vi "RANGE Write To File.vi"(6 "Time":dbl, 8 "Error In":errorcluster, 9 "All Meter Data":T2={"Meter 1"={"Meter Size"=0.0, "DAQ Output (Voltage)"=0.0, "Reference (Voltage)"=0.0, "Meter Present"=FALSE, "Meter Visa"="COM3", "Gas Type"="", "SLPM Error @ Zero"=0.0, "Gas Mix Number"="", "Set STP Register"=FALSE, "Measurement Units"={"Abs. Pressure"="", "Gauge/Diff. Press."="", "Barometric Press."="", "Temperature"="", "Volume"="", "Mass"="", "Setpoint"="", "Valve Drive"="", "Totalizer"="", "Tot. Timer"="", "Tot. Avg. Flow"="", "Tot. Peak Flow"="", "Software Version"=""}}, "Meter 2"={"Meter Size"=0.0, "DAQ Output (Voltage)"=0.0, "Reference (Voltage)"=0.0, "Meter Present"=FALSE, "Meter Visa"="COM3", "Gas Type"="", "SLPM Error @ Zero"=0.0, "Gas Mix Number"="", "Set STP Register"=FALSE, "Measurement Units"={"Abs. Pressure"="", "Gauge/Diff. Press."="", "Barometric Press."="", "Temperature"="", "Volume"="", "Mass"="", "Setpoint"="", "Valve Drive"="", "Totalizer"="", "Tot. Timer"="", "Tot. Avg. Flow"="", "Tot. Peak Flow"="", "Software Version"=""}}, "Meter 3"={"Meter Size"=0.0, "DAQ Output (Voltage)"=0.0, "Reference (Voltage)"=0.0, "Meter Present"=FALSE, "Meter Visa"="COM3", "Gas Type"="", "SLPM Error @ Zero"=0.0, "Gas Mix Number"="", "Set STP Register"=FALSE, "Measurement Units"={"Abs. Pressure"="", "Gauge/Diff. Press."="", "Barometric Press."="", "Temperature"="", "Volume"="", "Mass"="", "Setpoint"="", "Valve Drive"="", "Totalizer"="", "Tot. Timer"="", "Tot. Avg. Flow"="", "Tot. Peak Flow"="", "Software Version"=""}}, "Meter 4"={"Meter Size"=0.0, "DAQ Output (Voltage)"=0.0, "Reference (Voltage)"=0.0, "Meter Present"=FALSE, "Meter Visa"="COM3", "Gas Type"="", "SLPM Error @ Zero"=0.0, "Gas Mix Number"="", "Set STP Register"=FALSE, "Measurement Units"={"Abs. Pressure"="", "Gauge/Diff. Press."="", "Barometric Press."="", "Temperature"="", "Volume"="", "Mass"="", "Setpoint"="", "Valve Drive"="", "Totalizer"="", "Tot. Timer"="", "Tot. Avg. Flow"="", "Tot. Peak Flow"="", "Software Version"=""}}, "Meter 5"={"Meter Size"=0.0, "DAQ Output (Voltage)"=0.0, "Reference (Voltage)"=0.0, "Meter Present"=FALSE, "Meter Visa"="COM3", "Gas Type"="", "SLPM Error @ Zero"=0.0, "Gas Mix Number"="", "Set STP Register"=FALSE, "Measurement Units"={"Abs. Pressure"="", "Gauge/Diff. Press."="", "Barometric Press."="", "Temperature"="", "Volume"="", "Mass"="", "Setpoint"="", "Valve Drive"="", "Totalizer"="", "Tot. Timer"="", "Tot. Avg. Flow"="", "Tot. Peak Flow"="", "Software Version"=""}}, "Meter 6"={"Meter Size"=0.0, "DAQ Output (Voltage)"=0.0, "Reference (Voltage)"=0.0, "Meter Present"=FALSE, "Meter Visa"="COM3", "Gas Type"="", "SLPM Error @ Zero"=0.0, "Gas Mix Number"="", "Set STP Register"=FALSE, "Measurement Units"={"Abs. Pressure"="", "Gauge/Diff. Press."="", "Barometric Press."="", "Temperature"="", "Volume"="", "Mass"="", "Setpoint"="", "Valve Drive"="", "Totalizer"="", "Tot. Timer"="", "Tot. Avg. Flow"="", "Tot. Peak Flow"="", "Software Version"=""}}, "Meter Bank 1"={"Flow Rate (BTU/HR)"=0.0, "ANSI Placeholder Array"=[], "15 Sec Avg Array"=[], "30 Sec Avg Array "=[], "ANSI Average (BTU/HR)"=0.0, "Panel Data"={"Meter Type (Gas)"="", "Heating Value (BTU/ft³)"=0.0, "Ft³ / Hr (SCFH)"=0.0, "15 Second Average (BTU/HR)"=0.0, "30 Second Average (BTU/HR)"=0.0, "Mass Flow"=0.0, "Vol. Flow"=0.0, "Gas Temperature"=0.0, "Gas Pressure"=0.0, "Tot.Flow"=0.0}, "Start ANSI"=FALSE, "ANSI Start Time"=0.0, "Restart ANSI"=FALSE, "Meter ID"=""}, "Meter Bank 2"={"Flow Rate (BTU/HR)"=0.0, "ANSI Placeholder Array"=[], "15 Sec Avg Array"=[], "30 Sec Avg Array "=[], "ANSI Average (BTU/HR)"=0.0, "Panel Data"={"Meter Type (Gas)"="", "Heating Value (BTU/ft³)"=0.0, "Ft³ / Hr (SCFH)"=0.0, "15 Second Average (BTU/HR)"=0.0, "30 Second Average (BTU/HR)"=0.0, "Mass Flow"=0.0, "Vol. Flow"=0.0, "Gas Temperature"=0.0, "Gas Pressure"=0.0, "Tot.Flow"=0.0}, "Start ANSI"=FALSE, "ANSI Start Time"=0.0, "Restart ANSI"=FALSE, "Meter ID"=""}, "Meter Bank 3"={"Flow Rate (BTU/HR)"=0.0, "ANSI Placeholder Array"=[], "15 Sec Avg Array"=[], "30 Sec Avg Array "=[], "ANSI Average (BTU/HR)"=0.0, "Panel Data"={"Meter Type (Gas)"="", "Heating Value (BTU/ft³)"=0.0, "Ft³ / Hr (SCFH)"=0.0, "15 Second Average (BTU/HR)"=0.0, "30 Second Average (BTU/HR)"=0.0, "Mass Flow"=0.0, "Vol. Flow"=0.0, "Gas Temperature"=0.0, "Gas Pressure"=0.0, "Tot.Flow"=0.0}, "Start ANSI"=FALSE, "ANSI Start Time"=0.0, "Restart ANSI"=FALSE, "Meter ID"=""}, "Threshold Voltage (NI DAQ)"=0.2, "Use RS232 Data Collection"=FALSE, "Use Auto Switching"=FALSE}, 11 "File Path":path) -> (0 "Error Out":errorcluster)   [LabVIEW 2016]
uses:
  Type Definitions/RANGE DAQ Data Four Meters.ctl
  Type Definitions/RANGE DAQ Data.ctl
  Drivers/Omega FMA-1600A Series Gas Flow Meter/Type Definitions/FMA1600A Gas Type.ctl
  Drivers/Omega FMA-1600A Series Gas Flow Meter/Type Definitions/FMA1600A Units String.ctl
  Type Definitions/RANGE GAS Data.ctl
  Type Definitions/RANGE Panel Data.ctl
  <vilib>/Utility/file.llb/Write Delimited Spreadsheet (string).vi
panel:
  out "Debug":T1[](array[typedef])
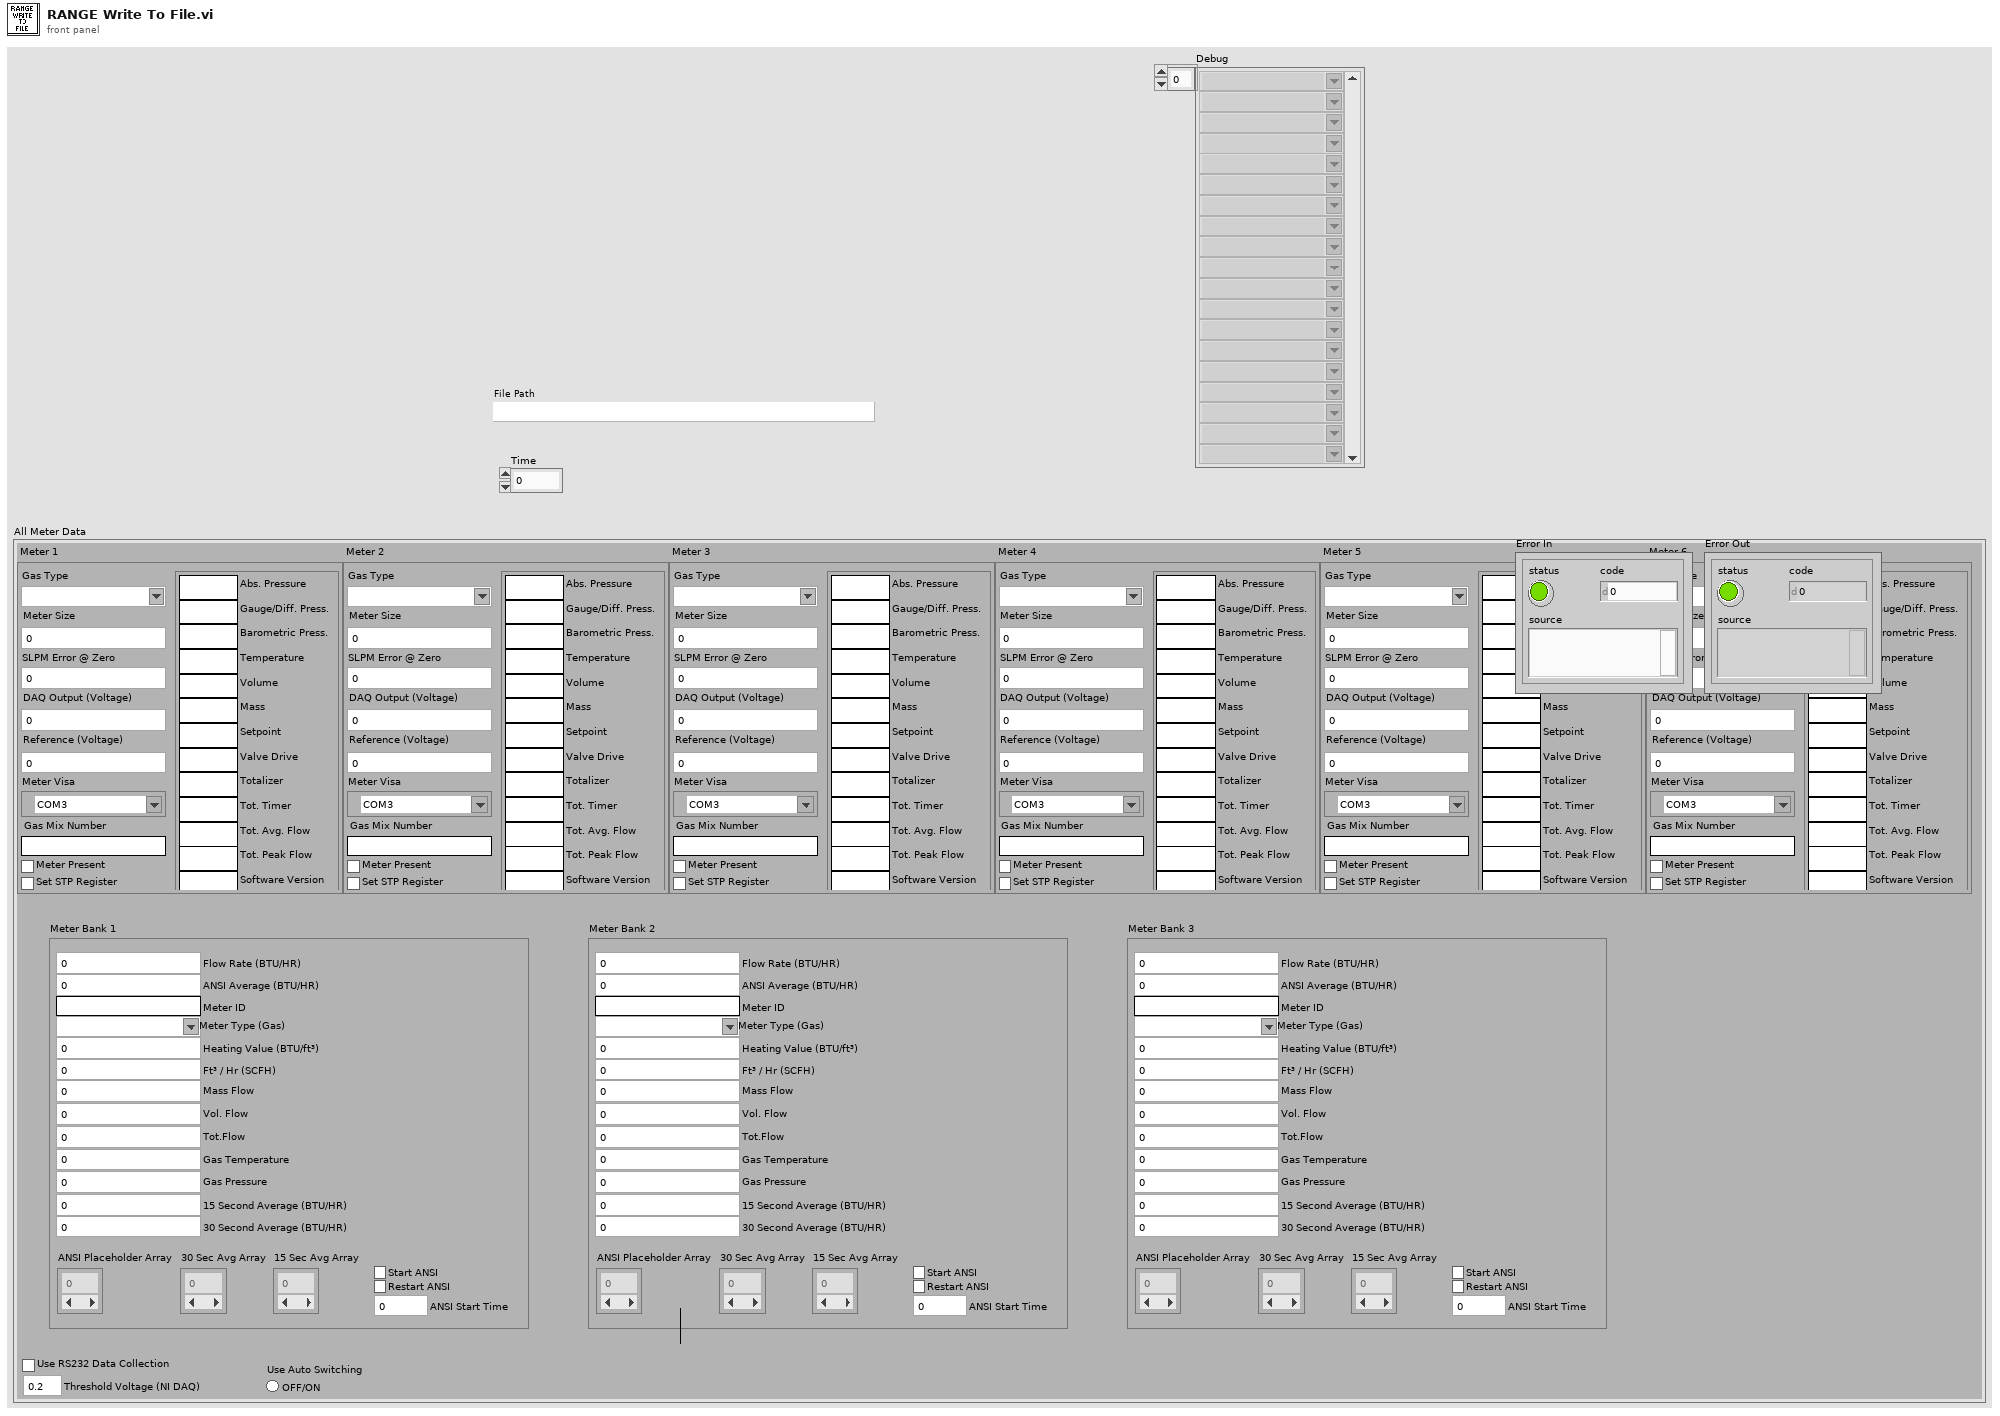
[diagram p1: front panel]
types:
  T1 = typedef "FMA1600A Gas Type.ctl" = string
  T2 = typedef "RANGE DAQ Data Four Meters.ctl" = cluster{"Meter 1":T3, "Meter 2":T3, "Meter 3":T3, "Meter 4":T3, "Meter 5":T3, "Meter 6":T3, "Meter Bank 1":T5, "Meter Bank 2":T5, "Meter Bank 3":T5, "Threshold Voltage (NI DAQ)":dbl, "Use RS232 Data Collection":bool, "Use Auto Switching":bool}
  T3 = typedef "RANGE DAQ Data.ctl" = cluster{"Meter Size":dbl, "DAQ Output (Voltage)":dbl, "Reference (Voltage)":dbl, "Meter Present":bool, "Meter Visa":refnum<visa-resource-name>, "Gas Type":T1, "SLPM Error @ Zero":dbl, "Gas Mix Number":string, "Set STP Register":bool, "Measurement Units":T4}
  T4 = typedef "FMA1600A Units String.ctl" = cluster{"Abs. Pressure":string, "Gauge/Diff. Press.":string, "Barometric Press.":string, "Temperature":string, "Volume":string, "Mass":string, "Setpoint":string, "Valve Drive":string, "Totalizer":string, "Tot. Timer":string, "Tot. Avg. Flow":string, "Tot. Peak Flow":string, "Software Version":string}
  T5 = typedef "RANGE GAS Data.ctl" = cluster{"Flow Rate (BTU/HR)":dbl, "ANSI Placeholder Array":dbl[], "15 Sec Avg Array":dbl[], "30 Sec Avg Array ":dbl[], "ANSI Average (BTU/HR)":dbl, "Panel Data":T6, "Start ANSI":bool, "ANSI Start Time":dbl, "Restart ANSI":bool, "Meter ID":string}
  T6 = typedef "RANGE Panel Data.ctl" = cluster{"Meter Type (Gas)":T1, "Heating Value (BTU/ft³)":dbl, "Ft³ / Hr (SCFH)":dbl, "15 Second Average (BTU/HR)":dbl, "30 Second Average (BTU/HR)":dbl, "Mass Flow":dbl, "Vol. Flow":dbl, "Gas Temperature":dbl, "Gas Pressure":dbl, "Tot.Flow":dbl}
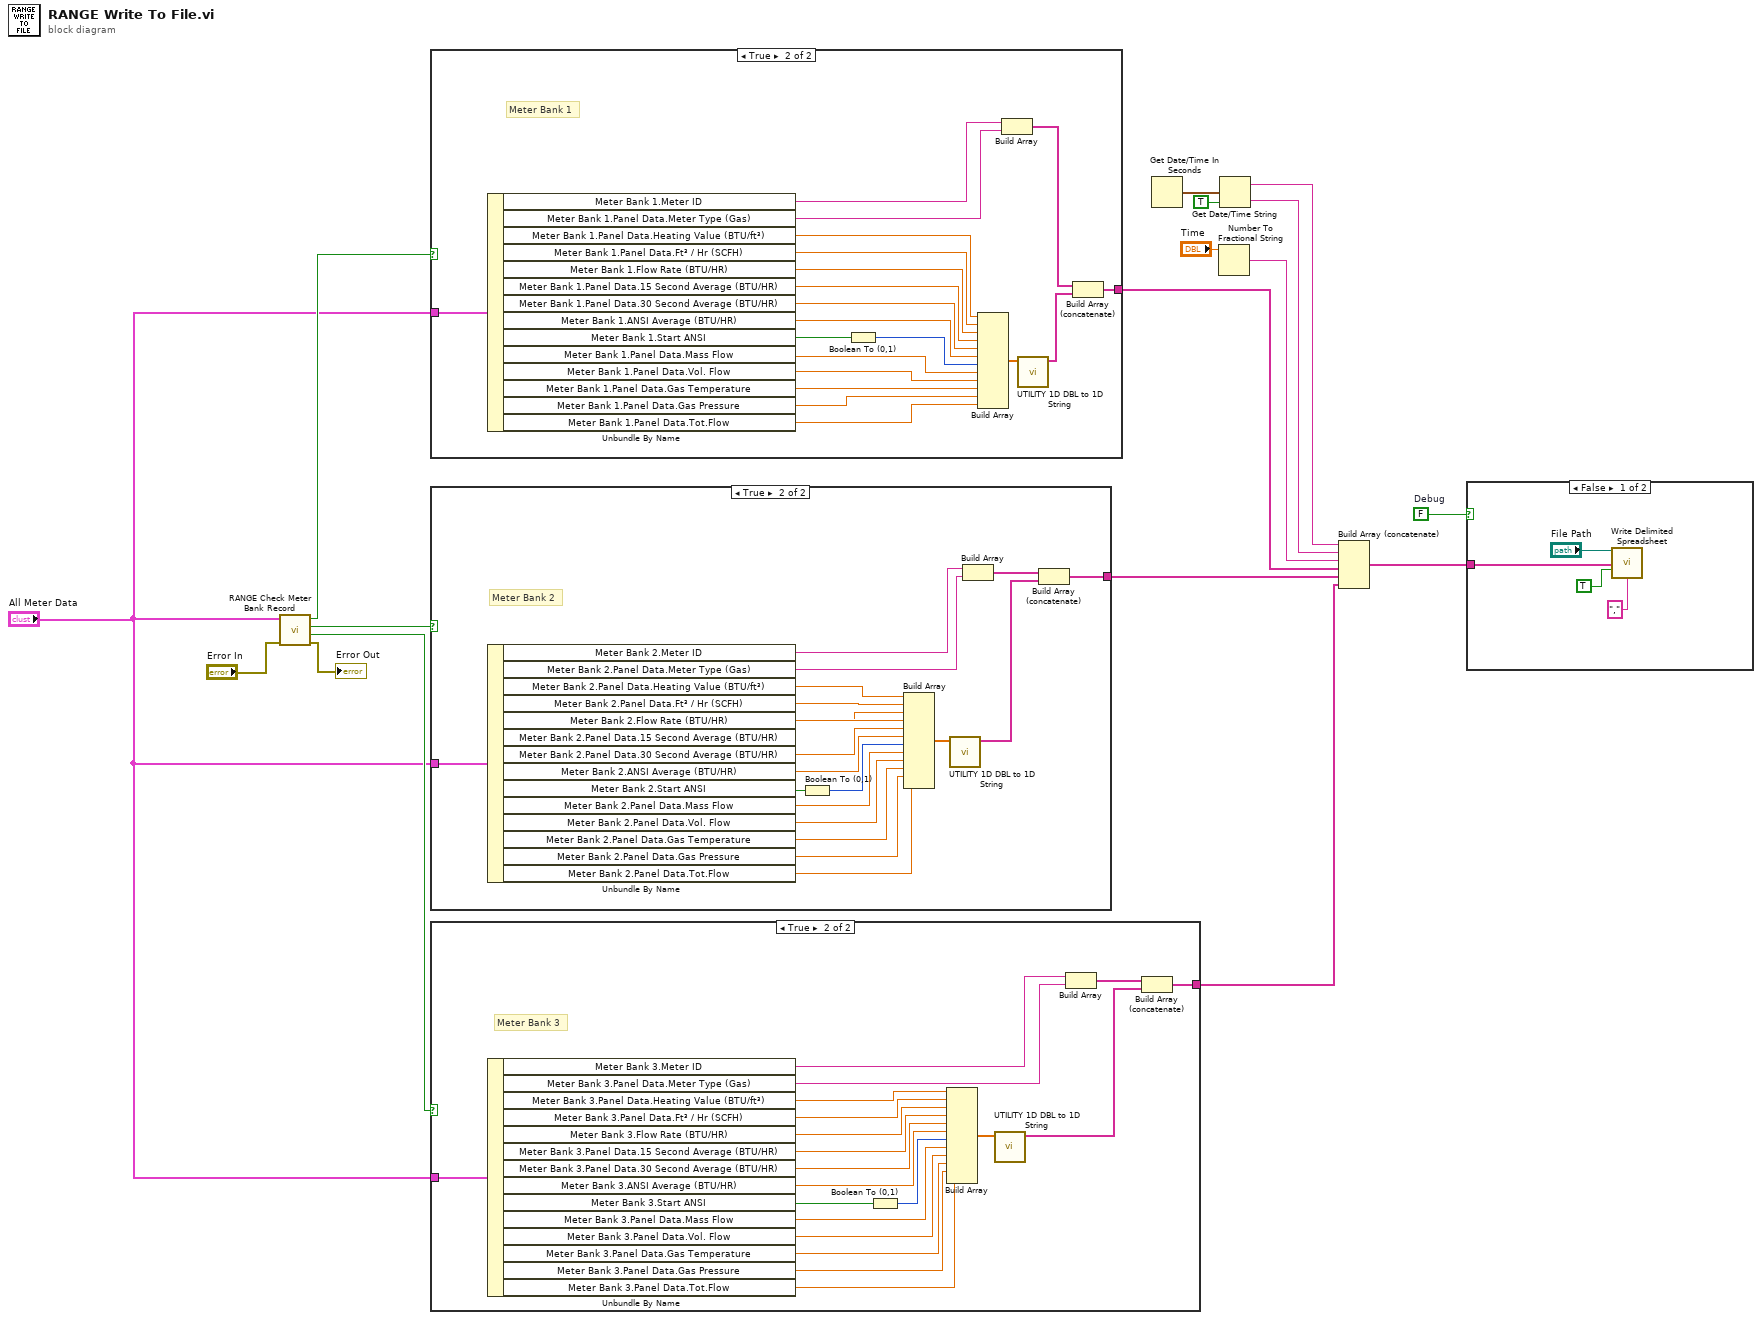
[diagram p0: block diagram]
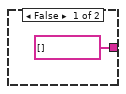
[diagram p2: hidden frame]
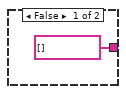
[diagram p3: hidden frame]
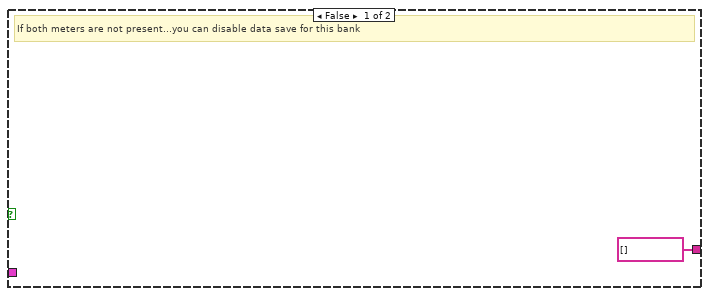
[diagram p4: hidden frame]
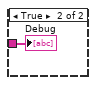
[diagram p5: hidden frame]
diagram:
  w7 = FALSE  # Debug
  n1 = call "RANGE Check Meter Bank Record.vi"("Error In"="Error In", "All Meter Data"="All Meter Data") -> ("Error Out"=→"Error Out":errorcluster, "Meter Bank 3"=w4:bool, "Meter Bank 2"=w5:bool, "Meter Bank 1"=w6:bool)  [unwired: 6 in]
  n2 = case shown="True" w6 {
    tunnel: "All Meter Data" -> [_ w31]
    tunnel: [T1[] [] w21] -> w15
    frame False {
      # "If both meters are not present...you can disable data save for this bank"
    }
    frame True {
      # "Meter Bank 1"
      n3 = Unbundle By Name(w31) -> ("Meter Bank 1.Meter ID"=w19:string, "Meter Bank 1.Panel Data.Meter Type (Gas)"=w24:T1, "Meter Bank 1.Panel Data.Heating Value (BTU/ft³)"=w38:dbl, "Meter Bank 1.Panel Data.Ft³ / Hr (SCFH)"=w37:dbl, "Meter Bank 1.Flow Rate (BTU/HR)"=w36:dbl, "Meter Bank 1.Panel Data.15 Second Average (BTU/HR)"=w35:dbl, "Meter Bank 1.Panel Data.30 Second Average (BTU/HR)"=w34:dbl, "Meter Bank 1.ANSI Average (BTU/HR)"=w33:dbl, "Meter Bank 1.Start ANSI"=w30:bool, "Meter Bank 1.Panel Data.Mass Flow"=w29:dbl, "Meter Bank 1.Panel Data.Vol. Flow"=w28:dbl, "Meter Bank 1.Panel Data.Gas Temperature"=w27:dbl, "Meter Bank 1.Panel Data.Gas Pressure"=w26:dbl, "Meter Bank 1.Panel Data.Tot.Flow"=w20:dbl)
      n4 = Boolean To (0,1)(Boolean=w30) -> (0, 1=w32:i16)
      n5 = Build Array(w38, w37, w36, w35, w34, w33, w32, w29, w28, w27, w26, w20) -> (w25:dbl[])
      n6 = Build Array(w19, w24) -> (w22:T1[])
      n7 = call "UTILITY 1D DBL to 1D String.vi"("1D DBL"=w25) -> ("1D String"=w23:string[])  [unwired: 10 in]
      n8 = Build Array (concatenate)(w22, w23) -> (w21:T1[])
    }
  }
  n9 = case shown="True" w5 {
    tunnel: [T1[] [] w43] -> w14
    tunnel: "All Meter Data" -> [_ w41]
    frame False {
    }
    frame True {
      # "Meter Bank 2"
      n10 = Unbundle By Name(w41) -> ("Meter Bank 2.Meter ID"=w40:string, "Meter Bank 2.Panel Data.Meter Type (Gas)"=w46:T1, "Meter Bank 2.Panel Data.Heating Value (BTU/ft³)"=w54:dbl, "Meter Bank 2.Panel Data.Ft³ / Hr (SCFH)"=w55:dbl, "Meter Bank 2.Flow Rate (BTU/HR)"=w56:dbl, "Meter Bank 2.Panel Data.15 Second Average (BTU/HR)"=w57:dbl, "Meter Bank 2.Panel Data.30 Second Average (BTU/HR)"=w58:dbl, "Meter Bank 2.ANSI Average (BTU/HR)"=w59:dbl, "Meter Bank 2.Start ANSI"=w52:bool, "Meter Bank 2.Panel Data.Mass Flow"=w51:dbl, "Meter Bank 2.Panel Data.Vol. Flow"=w50:dbl, "Meter Bank 2.Panel Data.Gas Temperature"=w49:dbl, "Meter Bank 2.Panel Data.Gas Pressure"=w48:dbl, "Meter Bank 2.Panel Data.Tot.Flow"=w42:dbl)
      n11 = Boolean To (0,1)(Boolean=w52) -> (0, 1=w53:i16)
      n12 = Build Array(w54, w55, w56, w57, w58, w59, w53, w51, w50, w49, w48, w42) -> (w47:dbl[])
      n13 = call "UTILITY 1D DBL to 1D String.vi"("1D DBL"=w47) -> ("1D String"=w45:string[])  [unwired: 10 in]
      n14 = Build Array(w40, w46) -> (w44:T1[])
      n15 = Build Array (concatenate)(w44, w45) -> (w43:T1[])
    }
  }
  n16 = case shown="True" w4 {
    tunnel: [T1[] [] w64] -> w13
    tunnel: "All Meter Data" -> [_ w62]
    frame False {
    }
    frame True {
      # "Meter Bank 3"
      n17 = Unbundle By Name(w62) -> ("Meter Bank 3.Meter ID"=w61:string, "Meter Bank 3.Panel Data.Meter Type (Gas)"=w66:T1, "Meter Bank 3.Panel Data.Heating Value (BTU/ft³)"=w80:dbl, "Meter Bank 3.Panel Data.Ft³ / Hr (SCFH)"=w79:dbl, "Meter Bank 3.Flow Rate (BTU/HR)"=w78:dbl, "Meter Bank 3.Panel Data.15 Second Average (BTU/HR)"=w77:dbl, "Meter Bank 3.Panel Data.30 Second Average (BTU/HR)"=w76:dbl, "Meter Bank 3.ANSI Average (BTU/HR)"=w75:dbl, "Meter Bank 3.Start ANSI"=w73:bool, "Meter Bank 3.Panel Data.Mass Flow"=w72:dbl, "Meter Bank 3.Panel Data.Vol. Flow"=w71:dbl, "Meter Bank 3.Panel Data.Gas Temperature"=w70:dbl, "Meter Bank 3.Panel Data.Gas Pressure"=w69:dbl, "Meter Bank 3.Panel Data.Tot.Flow"=w63:dbl)
      n18 = Boolean To (0,1)(Boolean=w73) -> (0, 1=w74:i16)
      n19 = Build Array(w80, w79, w78, w77, w76, w75, w74, w72, w71, w70, w69, w63) -> (w68:dbl[])
      n20 = call "UTILITY 1D DBL to 1D String.vi"("1D DBL"=w68) -> ("1D String"=w65:string[])  [unwired: 10 in]
      n21 = Build Array(w61, w66) -> (w67:T1[])
      n22 = Build Array (concatenate)(w67, w65) -> (w64:T1[])
    }
  }
  n23 = Get Date/Time In Seconds() -> (seconds since 1Jan1904=w12:timestamp)
  n24 = Number To Fractional String(number="Time") -> (F-format string=w16:string)  [unwired: 3 in]
  n25 = Get Date/Time String(seconds (now)=w12, want seconds? (F)=TRUE) -> (date string=w9:string, time string=w10:string)  [unwired: 1 in]
  n26 = Build Array (concatenate)(w9, w10, w16, w15, w14, w13) -> (w8:T1[])
  n27 = case shown="False" w7 {
    tunnel: w8 -> [w81 w85]
    frame False {
      n28 = call-poly <vilib>:"Write Delimited Spreadsheet.vi"("file path (dialog if empty)"="File Path", "1D data"=w81, "append to file? (new file:F)"=TRUE, "delimiter (\\t)"="," ("delimiter (\\t)")) -> ()  [unwired: 10 in, 2 out]
    }
    frame True {
      "Debug" <- w85
    }
  }
